vi "DT_Triangle Manager_Format Edge_Single Side.vi"(5 "left bottom tri":i32, 7 "left top tri":i32, 9 "start triangle":i32, 10 "right point":i32, 11 "left point":i32) -> (2 "Second Triangle":i32[](array[numeric]), 3 "First Triangle":i32[](array[numeric]))   [LabVIEW 2020, in "NI_AAL_Geometry.lvlib"]
uses:
  <vilib>/Analysis/NI_AAL_Geometry.lvlib
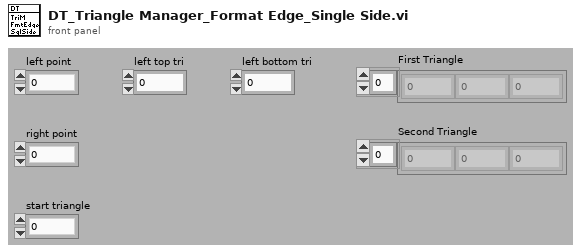
[diagram p1: front panel]
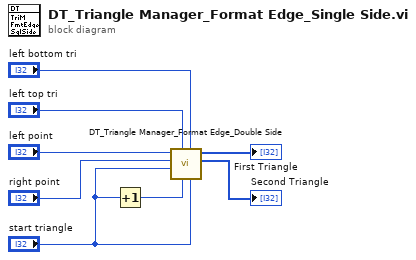
[diagram p0: block diagram]
diagram:
  n1 = Increment(x="start triangle") -> (x+1=w2:i32)
  n2 = call <vilib>:"DT_Triangle Manager_Format Edge_Double Side.vi"("right bottom tri"="start triangle", "left bottom tri"="left bottom tri", "right top tri"=w2, "left top tri"="left top tri", "start triangle"="start triangle", "right point"="right point", "left point"="left point") -> ("Second Triangle"=→"Second Triangle":i32[], "First Triangle"=→"First Triangle":i32[])  [unwired: 3 out]
